vi "GetDifferentiationProperties.vi"(8 "error in (no error)":errorcluster, 9 "Channels":T3[](array[typedef]), 10 "Channel Properties":T4[](array[typedef]), 11 "ChannelType":string) -> (0 "error out":errorcluster, 2 "Parent Channel Name":string, 3 "Differentiation Properties":T1={"Conversion Op"=enum."singleInt", "Unit"="", "Parent Unit"=""})   [LabVIEW 2017, in "CmsVirtualChannel.lvlib"]
uses:
  <vilib>/addons/InsightCM/Devices/Shared/Cms/CmsVirtualChannel/CmsVirtualChannel.lvlib
  <vilib>/addons/InsightCM/MessageBus/Base/controls/KeyValuePair.ctl
  <vilib>/addons/InsightCM/MessageBus/Base/controls/R2_Channel.ctl
  <vilib>/addons/InsightCM/MessageBus/Base/controls/Metric.ctl
  <vilib>/addons/InsightCM/Devices/Shared/Cms/CmsVirtualChannel/controls/Differentiation.ctl
  <vilib>/addons/InsightCM/Utilities/Analysis/Shared/controls/ConversionOp.ctl
  <vilib>/addons/InsightCM/Utilities/PropertyHelpers/PropertyHelpers.lvlib
  <vilib>/addons/InsightCM/Utilities/DeviceModelHelpers/DeviceModelHelpers.lvlib
  <vilib>/addons/InsightCM/Utilities/Analysis/Shared/AnalysisHelper.lvlib
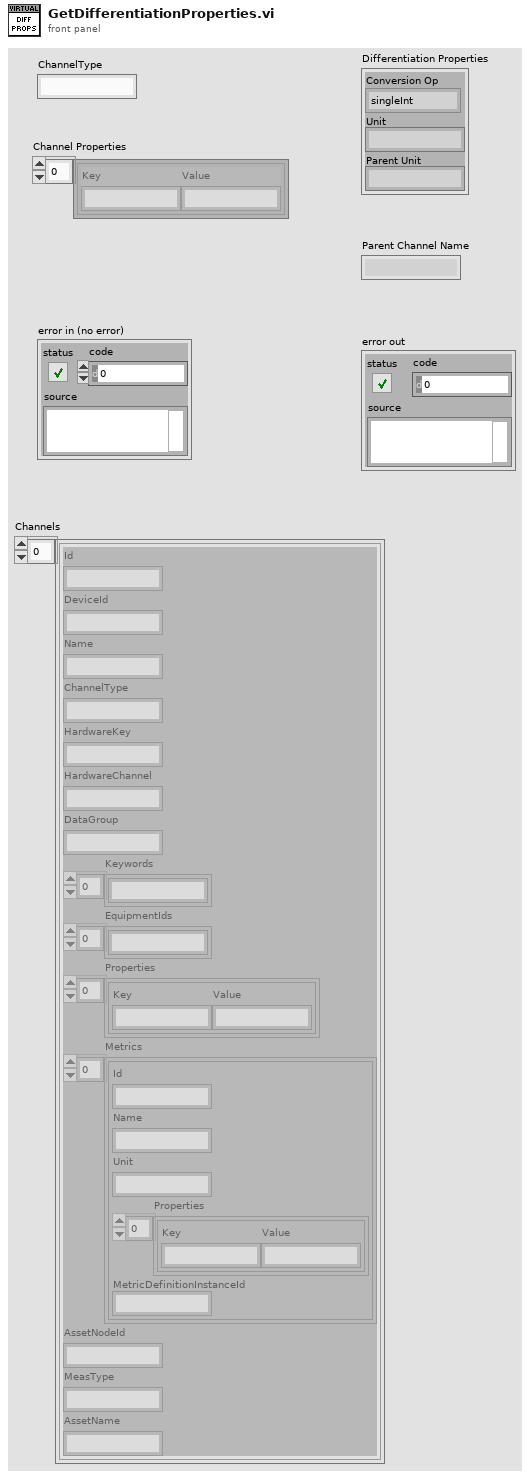
[diagram p1: front panel]
types:
  T1 = typedef "CmsVirtualChannel.lvlib/Differentiation.ctl" = cluster{"Conversion Op":T2, "Unit":string, "Parent Unit":string}
  T2 = typedef "AnalysisHelper.lvlib/ConversionOp.ctl" = enum16{"none", "singleInt", "doubleInt", "singleDiff", "doubleDiff"}
  T3 = typedef "R2_Channel.ctl" = cluster{"Id":string, "DeviceId":string, "Name":string, "ChannelType":string, "HardwareKey":string, "HardwareChannel":string, "DataGroup":string, "Keywords":string[], "EquipmentIds":string[], "Properties":T4[], "Metrics":T5[], "AssetNodeId":string, "MeasType":string, "AssetName":string}
  T4 = typedef "KeyValuePair.ctl" = cluster{"Key":string, "Value":string}
  T5 = typedef "Metric.ctl" = cluster{"Id":string, "Name":string, "Unit":string, "Properties":T4[], "MetricDefinitionInstanceId":string}
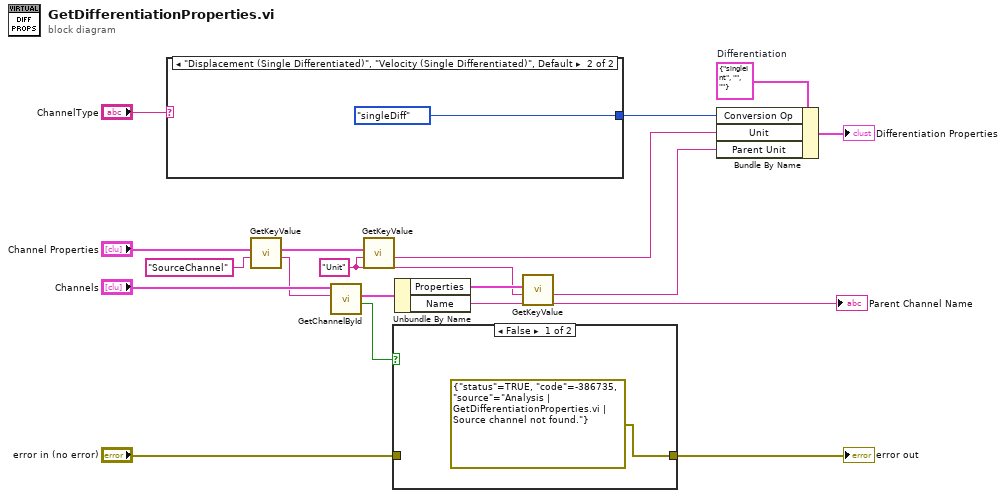
[diagram p0: block diagram]
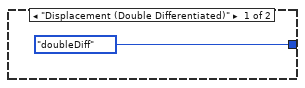
[diagram p2: hidden frame]
diagram:
  w2 = "Unit" ("key")
  w11 = T1 {"Conversion Op"=enum."singleInt", "Unit"="", "Parent Unit"=""}  # Differentiation
  n1 = case shown="\"Displacement (Single Differentiated)\", \"Velocity (Single Differentiated)\", Default" "ChannelType" {
    tunnel: [ConversionOp."doubleDiff" ("Conversion Op") ConversionOp."singleDiff" ("Conversion Op")] -> w9
    frame "Displacement (Double Differentiated)" {
    }
    frame "Displacement (Single Differentiated)", "Velocity (Single Differentiated)", Default {
    }
  }
  n2 = call <vilib>:"GetKeyValue.vi"("key"="SourceChannel" ("name"), "key value pairs"="Channel Properties") -> ("value"=w3:string, "key value pairs out"=w4:T4[])  [unwired: 7 in, 1 out]
  n3 = call <vilib>:"GetChannelById.vi"("channel id"=w3, "channels in"="Channels") -> ("found"=w16:bool, "channel"=w15:T3)  [unwired: 7 in, 1 out]
  n4 = call <vilib>:"GetKeyValue.vi"("key"=w2, "key value pairs"=w4) -> ("value"=w1:string)  [unwired: 7 in, 2 out]
  n5 = case shown="False" w16 {
    tunnel: [errorcluster {"status"=TRUE, "code"=-386735, "source"="Analysis | GetDifferentiationProperties.vi | Source channel not found."} ("error in (no error)") w22] -> w13
    tunnel: "error in (no error)" -> [_ w22]
    frame False {
    }
    frame True {
    }
  }
  "error out" <- w13
  n6 = Unbundle By Name(w15) -> ("Properties"=w7:T4[], "Name"=→"Parent Channel Name":string)
  n7 = call <vilib>:"GetKeyValue.vi"("key"=w2, "key value pairs"=w7) -> ("value"=w8:string)  [unwired: 7 in, 2 out]
  n8 = Bundle By Name(cluster=w11, "Conversion Op"=w9, "Unit"=w1, "Parent Unit"=w8) -> (→"Differentiation Properties":T1)
